vi "avToShortScalarAv.vi"(1 "attribute value":T1={"device name"="", "attribute name"="", "quality value"=0, "quality string"="", "timestamp"=0.0, "dim. x"=0, "dim. y"=0, "value"=[], "error code"=0, "error stack"=[], "data type"=36}) -> (0 "av":T2={"device name"="", "attribute name"="", "quality value"=0, "quality string"="", "timestamp"=0.0, "dim. x"=0, "dim. y"=0, "value"=0, "error code"=0, "error stack"=[], "data type"=36})   [LabVIEW 2014, in "tango.lvlib"]
uses:
  tango.lvlib
  base/toShortScalar.vi
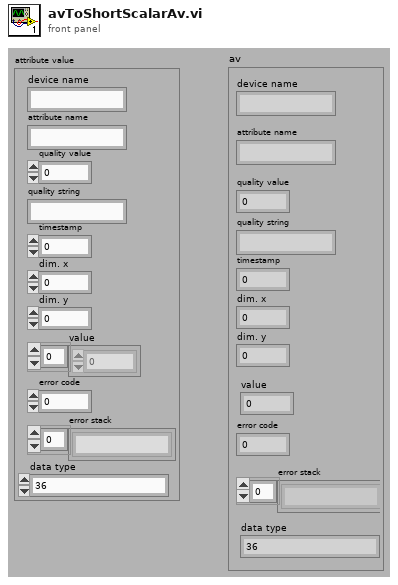
[diagram p1: front panel]
types:
  T1 = cluster{"device name":string, "attribute name":string, "quality value":i16, "quality string":string, "timestamp":dbl, "dim. x":i32, "dim. y":i32, "value":u8[], "error code":i32, "error stack":string[], "data type":u16}
  T2 = cluster{"device name":string, "attribute name":string, "quality value":i16, "quality string":string, "timestamp":dbl, "dim. x":i32, "dim. y":i32, "value":i16, "error code":i32, "error stack":string[], "data type":u16}
  T3 = cluster{"device name":string, "attribute name":string, "quality value":i16, "quality string":string, "timestamp":dbl, "dim. x":i32, "dim. y":i32, "value_out":i16, "error code":i32, "error stack":string[], "data type":u16}
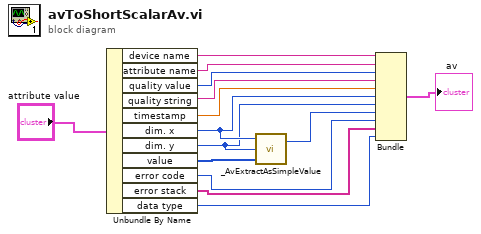
[diagram p0: block diagram]
diagram:
  n1 = Unbundle By Name("attribute value") -> ("device name"=w14:string, "attribute name"=w13:string, "quality value"=w12:i16, "quality string"=w11:string, "timestamp"=w10:dbl, "dim. x"=w4:i32, "dim. y"=w3:i32, "value"=w5:u8[], "error code"=w8:i32, "error stack"=w7:string[], "data type"=w1:u16)
  n2 = call-poly "_AvExtractAsSimpleValue.vi"("value_in"=w5, "dim_y"=w3, "dim_x"=w4) -> ("value_out"=w9:i16)  [unwired: 1 out]
  n3 = Bundle("device name"=w14, "attribute name"=w13, "quality value"=w12, "quality string"=w11, "timestamp"=w10, "dim. x"=w4, "dim. y"=w3, "value_out"=w9, "error code"=w8, "error stack"=w7, "data type"=w1) -> (→"av":T3)  [unwired: 1 in]
